vi "DigitalInOut_mode.vi"(8 "error in (no error)":errorcluster, 10 "PinMode":string, 11 "DigitalInOut in":refnum<class "DigitalInOut.lvclass">) -> (0 "error out":errorcluster, 3 "DigitalInOut out":refnum<class "DigitalInOut.lvclass">)   [LabVIEW 2011, in "mbed_LVLibrary.lvlib" / "DigitalInOut.lvclass"]
uses:
  DigitalInOut.lvclass
  DigitalInOut.lvclass/DigitalInOut.ctl
  Transport Mechanisms/mbed/mbed.lvclass
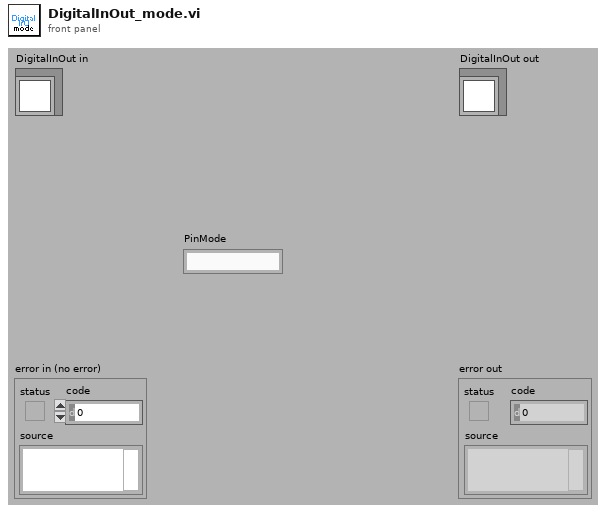
[diagram p1: front panel]
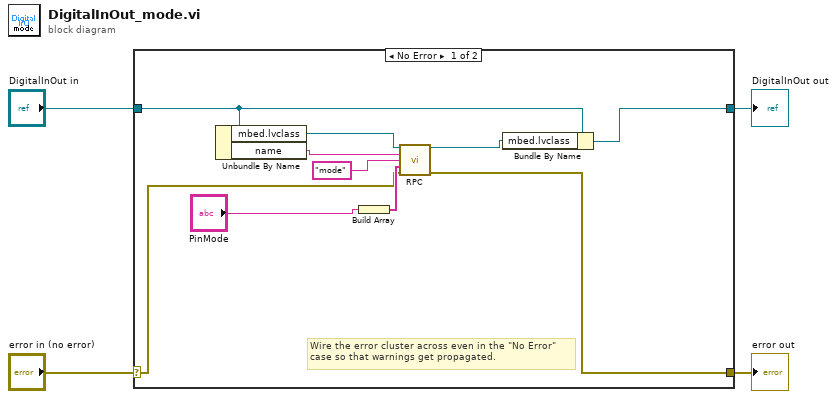
[diagram p0: block diagram]
diagram:
  n1 = case shown="No Error" "error in (no error)" {
    selector: "error in (no error)" -> [w7 w16]
    tunnel: [w6 w16] -> w3
    tunnel: [w8 w15] -> w1
    tunnel: "DigitalInOut in" -> [w14 w15]
    frame No Error {
      # "Wire the error cluster across even in the \"No Error\"\ncase so that warnings get propagated."
      n2 = Unbundle By Name(w14) -> ("mbed.lvclass"=w13:refnum<class "mbed.lvclass">, "name"=w11:string)
      n3 = Build Array("PinMode") -> (w9:string[])
      n4 = call-dynamic "RPC.vi"("mbed in"=w13, "Name"=w11, "method"="mode", "Args"=w9, "error in (no error)"=w7) -> ("mbed out"=w12:refnum<class "mbed.lvclass">, "error out"=w6:errorcluster)  [unwired: 8 in, 1 out]
      n5 = Bundle By Name(cluster=w14, "mbed.lvclass"=w12) -> (w8:refnum<class "DigitalInOut.lvclass">)
    }
    frame Error {
    }
  }
  "error out" <- w3
  "DigitalInOut out" <- w1
